vi "DUAL GAUGE-Get 2 Pressure,Status.vi"(8 "Fehler (Eingang)":errorcluster, 11 "Referenz in":refnum<visa-resource-name>) -> (0 "Cluster (Ausgang)":errorcluster, 1 "Pressure Sensor 2":dbl format="%.3e", 2 "Pressure Sensor 1":dbl format="%.3e", 3 "Referenz out":refnum<visa-resource-name>, 4 "Status Sensor 2":i32(ring) items=["data OK", "underrange", "overrange", "sensor error", "sensor off", "no sensor", "ID error"], 5 "Status Sensor 1":i32(ring) items=["data OK", "underrange", "overrange", "sensor error", "sensor off", "no sensor", "ID error"])   [LabVIEW 2017, in "Dual Gauge.lvlib"]
uses:
  <userlib>/Dual Gauge/Dual Gauge.lvlib
panel:
  # "mbar"
  # "mbar"
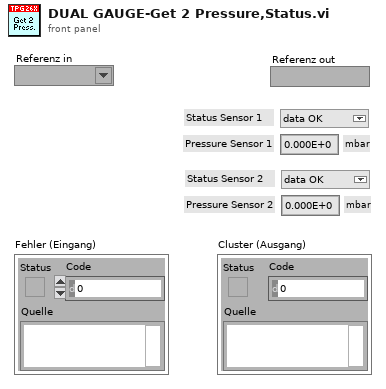
[diagram p1: front panel]
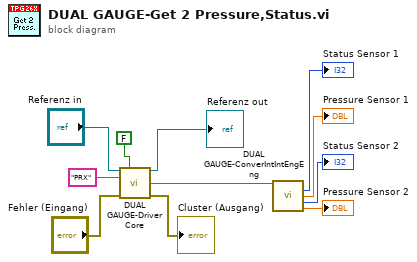
[diagram p0: block diagram]
diagram:
  n1 = call <userlib>:"DUAL GAUGE-Driver Core.vi"("Referenz in"="Referenz in", "Write/Read"=FALSE, "Command"="PRX", "Fehler (Eingang)"="Fehler (Eingang)") -> ("Referenz out"=→"Referenz out":refnum<visa-resource-name>, "String Out"=w6:string, "Cluster (Ausgang)"=→"Cluster (Ausgang)":errorcluster)  [unwired: 9 in]
  n2 = call <userlib>:"DUAL GAUGE-ConverIntIntEngEng.vi"("String in"=w6) -> ("Integer1 out"=→"Status Sensor 1":u8, "Eng1 out"=→"Pressure Sensor 1":dbl, "Integer2 out"=→"Status Sensor 2":u8, "Eng2 out"=→"Pressure Sensor 2":dbl)  [unwired: 11 in]
